vi "standard name.vi"(8 "error in":errorcluster, 9 "zero index bit":bool, 10 "zero index element":bool, 11 "Modbus Module Channel in":refnum<class "Modbus Module Channel.lvclass">) -> (0 "error out":errorcluster, 2 "standard name":string, 3 "Modbus Module Channel out":refnum<class "Modbus Module Channel.lvclass">)   [LabVIEW 2013, in "Modbus Module Channel.lvclass"]
uses:
  Modbus Module Channel.lvclass
  <vilib>/NI/Tag Bus/tag/Data Type.ctl
  Modbus Module Channel.lvclass/Modbus Module Channel.ctl
  <vilib>/NI/Tag Bus/tag/tag descriptor.lvclass/tag descriptor.ctl
  Read modbus type.vi
  Read starting address.vi
  <vilib>/NI/Tag Bus/tag/read data type.vi
  Read subindex (bool).vi
  <vilib>/NI/Tag Bus/tag/tag descriptor.lvclass
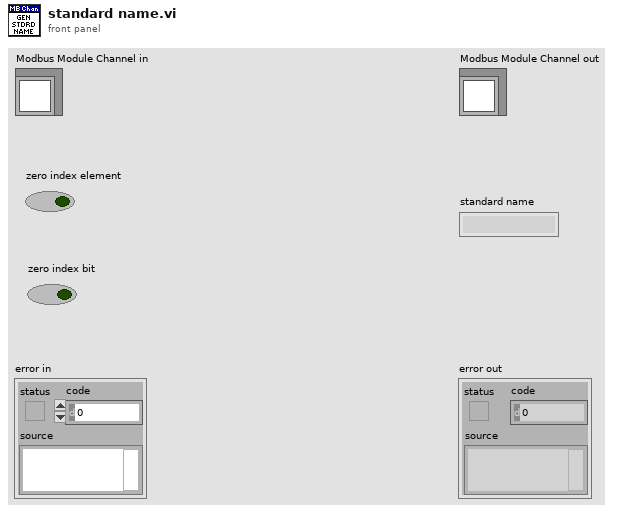
[diagram p1: front panel]
types:
  T1 = typedef "tag bus.lvlib/tag descriptor.lvclass/Data Type.ctl" = enum16{"Double", "Single", "I64", "I32", "I16", "I8", "U64", "U32", "U16", "U8", "Boolean", "String", "Array of Double", "Array of Single", "Array of I64", "Array of I32", "Array of I16", "Array of I8", "Array of U64", "Array of U32", "Array of U16", "Array of U8", "Array of Boolean", "Array of String"}
  T2 = typedef "Modbus Module Channel.lvclass/data bank type.ctl" = enum16{"coils", "discrete inputs", "input registers", "holding registers"}
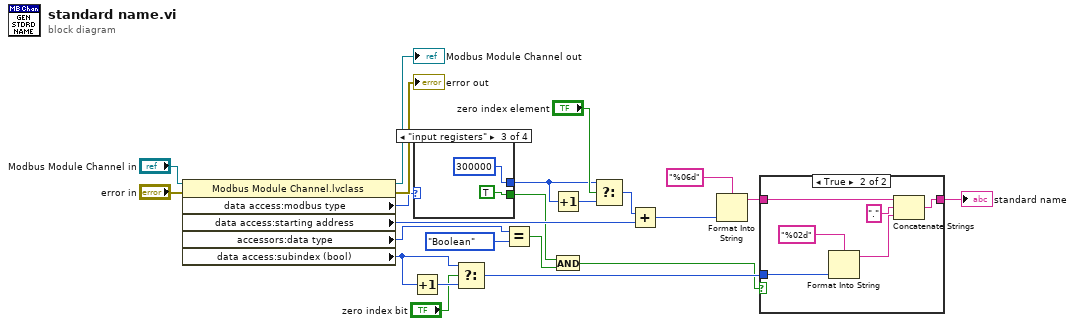
[diagram p0: block diagram]
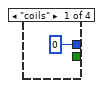
[diagram p3: hidden frame]
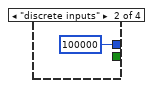
[diagram p4: hidden frame]
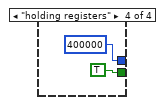
[diagram p5: hidden frame]
diagram:
  n1 = property class="Modbus Module Channel.lvclass"(reference="Modbus Module Channel in", error in="error in") -> (reference out=→"Modbus Module Channel out":refnum<class "Modbus Module Channel.lvclass">, error out=→"error out":errorcluster, "data access:modbus type"=w19:T2, "data access:starting address"=w14:u16, "accessors:data type"=w11:T1, "data access:subindex (bool)"=w7:i32)
  n2 = Increment(x=w7) -> (x+1=w9:i32)
  n3 = case shown="\"input registers\"" w19 {
    tunnel: [0 100000 300000 400000] -> w17
    tunnel: [_ _ TRUE TRUE] -> w13
    frame "coils" {
    }
    frame "discrete inputs" {
    }
    frame "input registers" {
    }
    frame "holding registers" {
    }
  }
  n4 = Select(t=w7, s="zero index bit", f=w9) -> (s? t:f=w6:i32)
  n5 = Equal?(x=w11, y=Data_Type."Boolean") -> (x = y?=w12:bool)
  n6 = Increment(x=w17) -> (x+1=w16:i32)
  n7 = And(x=w13, y=w12) -> (x .and. y?=w5:bool)
  n8 = Select(t=w17, s="zero index element", f=w16) -> (s? t:f=w15:i32)
  n9 = Add(x=w15, y=w14) -> (x+y=w3:i32)
  n10 = Format Into String(format string="%06d", w3) -> (resulting string=w2:string)  [unwired: 2 in, 1 out]
  n11 = case shown="True" w5 {
    tunnel: w6 -> [_ w33]
    tunnel: w2 -> [w30 w36]
    tunnel: [w30 w34] -> w4
    frame False {
    }
    frame True {
      n12 = Format Into String(format string="%02d", w33) -> (resulting string=w32:string)  [unwired: 2 in, 1 out]
      n13 = Concatenate Strings(w36, "." ("string"), w32) -> (w34:string)
    }
  }
  "standard name" <- w4
